vi "General LS Linear Fit.vi"(0 "Y":dbl[](array[numeric]) format="%0.2f", 5 "H":dbl[][](array[numeric]) format="%0.2f", 7 "Weight":dbl[](array[numeric]) format="%0.2f", 9 "covariance selector":T2(ring), 11 "algorithm":T1 items=["SVD", "Givens", "Givens2", "Householder", "LU Decomposition", "Cholesky", "SVD for Rank Deficient H"]) -> (4 "Best Fit":dbl[](array[numeric]) format="%0.2f", 6 "Coefficients":dbl[](array[numeric]) format="%0.2f", 8 "Covariance":T3, 14 "mse":dbl format="%0.2f", 15 "error":i32)   [LabVIEW 2017, in "NI_AALPro.lvlib"]
doc: "Finds the k-dimension linear curve values and the set of k-dimension linear fit coefficients, which describe the k-dimension linear curve that best represents the input data set using the least-squares solution."
uses:
  NI_AALPro.lvlib
  RealMatrix.ctl
  General Linear Fit Algorithm.ctl
  Array To Matrix - RA2.vi
  NI_Matrix.lvlib
  <resource>/lvanlys.dll
panel:
  # "General LS Linear Fit"
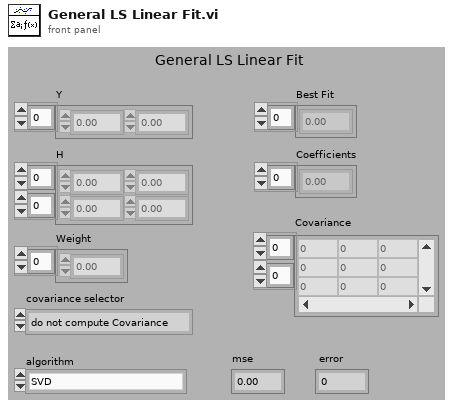
[diagram p1: front panel]
types:
  T1 = typedef "NI_AALPro.lvlib/General Linear Fit Algorithm.ctl" = u16
  T2 = enum32{"do not compute Covariance", " compute Covariance"}
  T3 = typedef "NI_Matrix.lvlib/RealMatrix.ctl" = dbl[][]
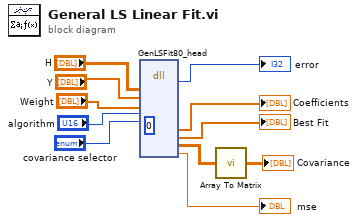
[diagram p0: block diagram]
diagram:
  (unwired) 0
  n1 = dll-call lib="C:/Program Files (x86)/National Instruments/LabVIEW 2017/resource/lvanlys.*" fn="GenLSFit80_head"("H"="H", "Y Values"="Y", "Weight"="Weight", "algorithm"="algorithm", "covariance selector"="covariance selector") -> ("return type"=→"error":i32, "CoefH"=→"Coefficients":dbl[], "BestFitH"=→"Best Fit":dbl[], "CovarH"=w3:dbl[][], "mse"=→"mse":dbl)  [unwired: 6 in, 8 out]
  n2 = call-poly "Array To Matrix.vi"("Real 2D Array"=w3) -> ("Real Matrix"=→"Covariance":T3)
